vi "Send Command.vi"(8 "error in (no error)":errorcluster, 10 "Register Address":u8 format="%.0x", 11 "LINX-ADS1256 in":refnum<class "LINX-ADS1256.lvclass">) -> (0 "error out":errorcluster, 3 "LINX-ADS1256 out":refnum<class "LINX-ADS1256.lvclass">)   [LabVIEW 2020, in "LINX-ADS1256.lvclass"]
uses:
  LINX-ADS1256.lvclass
  LINX SPI/LINX SPI.lvclass
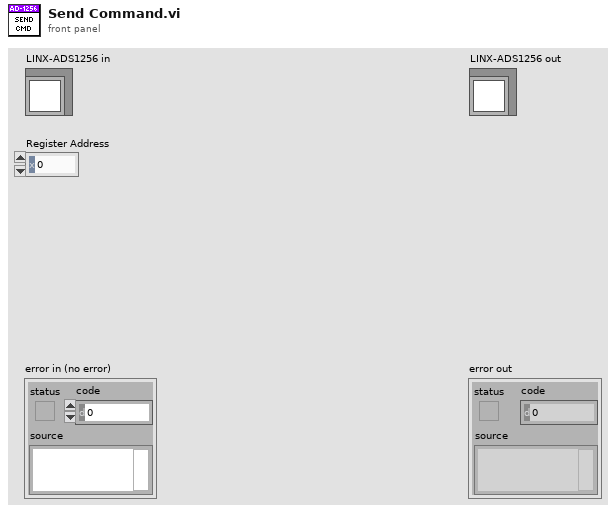
[diagram p1: front panel]
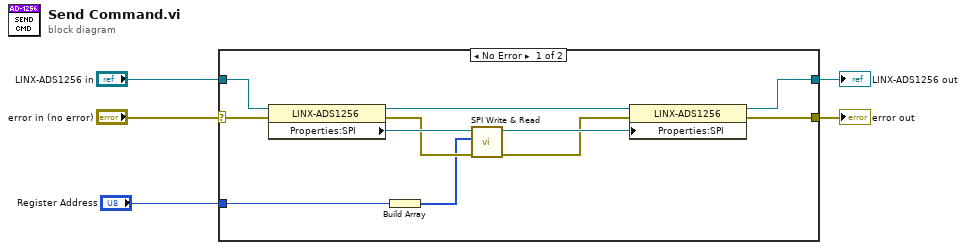
[diagram p0: block diagram]
diagram:
  n1 = case shown="No Error" "error in (no error)" {
    selector: "error in (no error)" -> [w9 w18]
    tunnel: [w8 w18] -> w4
    tunnel: [w10 w17] -> w2
    tunnel: "LINX-ADS1256 in" -> [w16 w17]
    tunnel: "Register Address" -> [w7 _]
    frame No Error {
      n2 = property class="LINX-ADS1256"(reference=w16, error in=w9) -> (reference out=w12:refnum<class "LINX-ADS1256.lvclass">, error out=w13:errorcluster, "Properties:SPI"=w15:refnum<class "LINX SPI.lvclass">)
      n3 = Build Array(w7) -> (w6:u8[])
      n4 = call "SPI Write & Read.vi"("error in (no error)"=w13, "Data"=w6, "LINX SPI in"=w15) -> ("error out"=w11:errorcluster, "LINX SPI out"=w14:refnum<class "LINX SPI.lvclass">)  [unwired: 6 in, 1 out]
      n5 = property class="LINX-ADS1256"(reference=w12, error in=w11, "Properties:SPI"=w14) -> (reference out=w10:refnum<class "LINX-ADS1256.lvclass">, error out=w8:errorcluster)
    }
    frame Error {
    }
  }
  "error out" <- w4
  "LINX-ADS1256 out" <- w2
